vi "MGI Position to Array Index.vi"(8 "error in (no error)":errorcluster, 10 "Coords":T2, 11 "ArrayRef":refnum<vi>) -> (0 "error out":errorcluster, 1 "Element Size":cluster{"Width":i32, "Height":i32}, 2 "Index":T1, 3 "ArrayRef (Dup)":refnum<vi>, 4 "In Bounds?":bool)   [LabVIEW 2020]
doc: "Outputs the Cell Position and Cell Bounds of the Array element containing the specified coordinates. If the coordinates are outside of the array control, <B>In Bounds?</B> is false. \n\nAuthored by Stephen Moore\nsupport@mooregoodideas.com\nwww.mooregoodideas.com\n\nCopyright (c) 2010, Moore Good Ideas, Inc.\n\nAll rights reserved.\n\nRedistribution and use in source and binary forms, with or without modification, are permitted provided that the following conditions are met:\n\n * Redistributions of source code must retain the above copyright notice, this list of conditions and the following disclaimer.\n * Redistributions in binary form must reproduce the above copyright notice, this list of conditions and the following disclaimer in the documentation and/or other materials provided with the distribution.\n * Neither the name of Moore Good Ideas, Inc. nor the names of its contributors may be used to endorse or promote products derived from this software without specific prior written permission.\n\nTHIS SOFTWARE IS PROVIDED BY THE COPYRIGHT HOLDERS AND CONTRIBUTORS \"AS IS\" AND ANY EXPRESS OR IMPLIED WARRANTIES, INCLUDING, BUT NOT LIMITED TO, THE IMPLIED WARRANTIES OF MERCHANTABILITY AND FITNESS FOR A PARTICULAR PURPOSE ARE DISCLAIMED. IN NO EVENT SHALL THE COPYRIGHT OWNER OR CONTRIBUTORS BE LIABLE FOR ANY DIRECT, INDIRECT, INCIDENTAL, SPECIAL, EXEMPLARY, OR CONSEQUENTIAL DAMAGES (INCLUDING, BUT NOT LIMITED TO, PROCUREMENT OF SUBSTITUTE GOODS OR SERVICES; LOSS OF USE, DATA, OR PROFITS; OR BUSINESS INTERRUPTION) HOWEVER CAUSED AND ON ANY THEORY OF LIABILITY, WHETHER IN CONTRACT, STRICT LIABILITY, OR TORT (INCLUDING NEGLIGENCE OR OTHERWISE) ARISING IN ANY WAY OUT OF THE USE OF THIS SOFTWARE, EVEN IF ADVISED OF THE POSSIBILITY OF SUCH DAMAGE."
uses:
  <vilib>/Utility/miscctls.llb/LVPoint32TypeDef.ctl
  <vilib>/Utility/miscctls.llb/LVRowAndColumnTypeDef.ctl
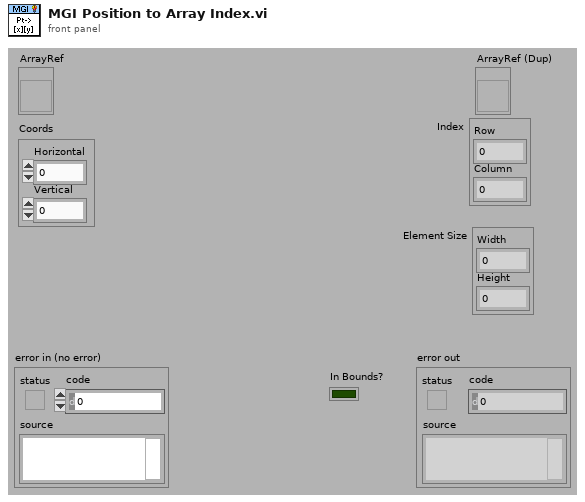
[diagram p1: front panel]
types:
  T1 = typedef "LVRowAndColumnTypeDef.ctl" = cluster{"Row":i32, "Column":i32}
  T2 = typedef "LVPoint32TypeDef.ctl" = cluster{"Horizontal":i32, "Vertical":i32}
  T3 = typedef "LVRectTypeDef.ctl" = cluster{"Left":i16, "Top":i16, "Right":i16, "Bottom":i16}
  T4 = typedef "LVBoundsTypeDef.ctl" = cluster{"Width":u32, "Height":u32}
  T5 = cluster{"Number of Columns":u32, "Number of Rows":u32}
  T6 = cluster{"Number of Columns":i32, "Number of Rows":i32}
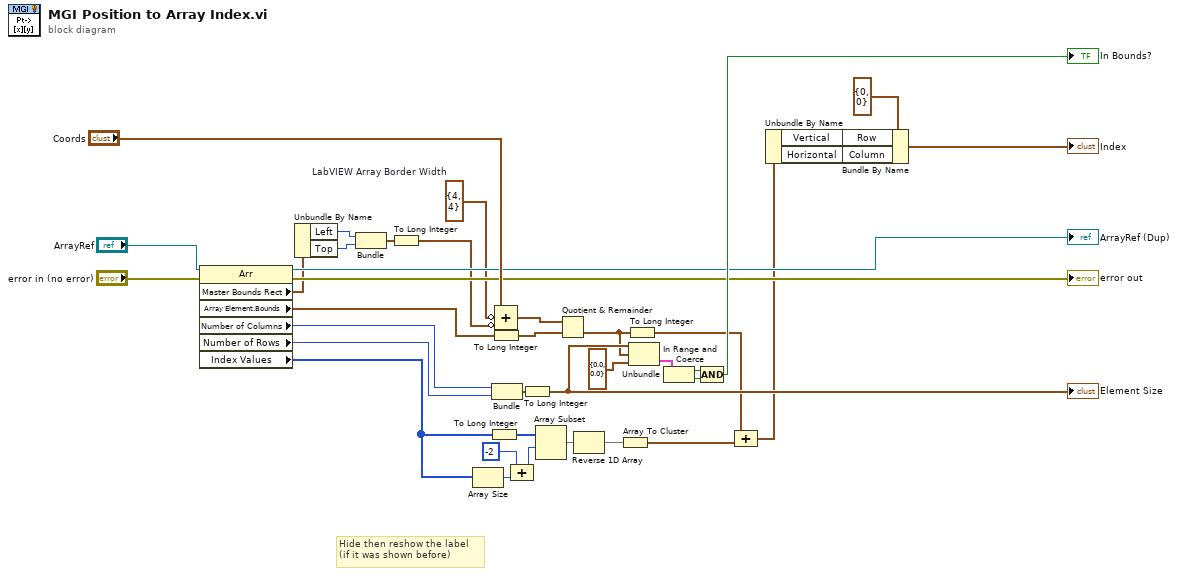
[diagram p0: block diagram]
diagram:
  w3 = T2 {"Horizontal"=4, "Vertical"=4}  # LabVIEW Array Border Width
  # "Hide then reshow the label \n(if it was shown before)"
  n1 = property on="Property Node" class="Arr"(reference="ArrayRef", error in="error in (no error)") -> (reference out=→"ArrayRef (Dup)":refnum<vi>, error out=→"error out":errorcluster, "Master Bounds Rect"=w8:T3, "Array Element.Bounds"=w9:T4, "Number of Columns"=w10:u32, "Number of Rows"=w11:u32, "Index Values"=w12:u32[])
  n2 = Unbundle By Name(w8) -> ("Left"=w6:i16, "Top"=w7:i16)
  n3 = Bundle("Left"=w6, "Top"=w7) -> (w5:cluster{"Left":i16, "Top":i16})  [unwired: 1 in]
  n4 = To Long Integer(number=w5) -> (32bit integer=w4:cluster{"Left":i32, "Top":i32})
  n5 = Array Size(array=w12) -> (size(s)=w23:i32)
  n6 = To Long Integer(number=w12) -> (32bit integer=w24:i32[])
  n7 = To Long Integer(number=w9) -> (32bit integer=w29:cluster{"Width":i32, "Height":i32})
  n8 = Bundle("Number of Columns"=w10, "Number of Rows"=w11) -> (w17:T5)  [unwired: 1 in]
  n9 = Compound Arithmetic op=ADD("Coords", invert w3, invert w4) -> (w28:T2)
  n10 = Compound Arithmetic op=ADD(-2 ("value"), w23) -> (w25:i32)
  n11 = To Long Integer(number=w17) -> (32bit integer=w36:T6)
  "Element Size" <- w36
  n12 = Array Subset(array=w24, index=w25) -> (w26:i32[])  [unwired: 1 in]
  n13 = Quotient & Remainder(x=w28, y=w29) -> (floor(x/y)=w30:T2)  [unwired: 1 out]
  n14 = Reverse 1D Array(array=w26) -> (reversed array=w1:i32[])
  n15 = Array To Cluster(array=w1) -> (cluster=w27:cluster{"[0]":i32, "[1]":i32})
  n16 = To Long Integer(number=w30) -> (32bit integer=w2:T2)
  n17 = In Range and Coerce(upper limit=w36, x=w30, lower limit=cluster{dbl, dbl} {0.0, 0.0}) -> (In Range?=w19:cluster{"Horizontal":bool, "Vertical":bool})  [unwired: 1 out]
  n18 = Unbundle(w19) -> ("Horizontal"=w20:bool, "Vertical"=w21:bool)
  n19 = Compound Arithmetic op=AND(w20, w21) -> (→"In Bounds?":bool)
  n20 = Compound Arithmetic op=ADD(w2, w27) -> (w15:T2)
  n21 = Unbundle By Name(w15) -> ("Vertical"=w14:i32, "Horizontal"=w13:i32)
  n22 = Bundle By Name(cluster=T1 {"Row"=0, "Column"=0} ("Cell Position"), "Row"=w14, "Column"=w13) -> (→"Index":T1)
